vi "水样测试配置.vi"() -> (2 "确认输出":bool, 3 "水样测定时间输出":dbl=1.0)   [LabVIEW 2016, in "斯坦道多参数.lvlib"]
uses:
  <vilib>/Utility/config.llb/NI_LVConfig.lvlib
  <vilib>/Utility/miscctls.llb/LVPointTypeDef.ctl
panel:
  in  "取消":bool
  in  "确定":bool
  in  "水样测试时间":dbl=1.0
  # "请输入水样测定时间"
  # "min"
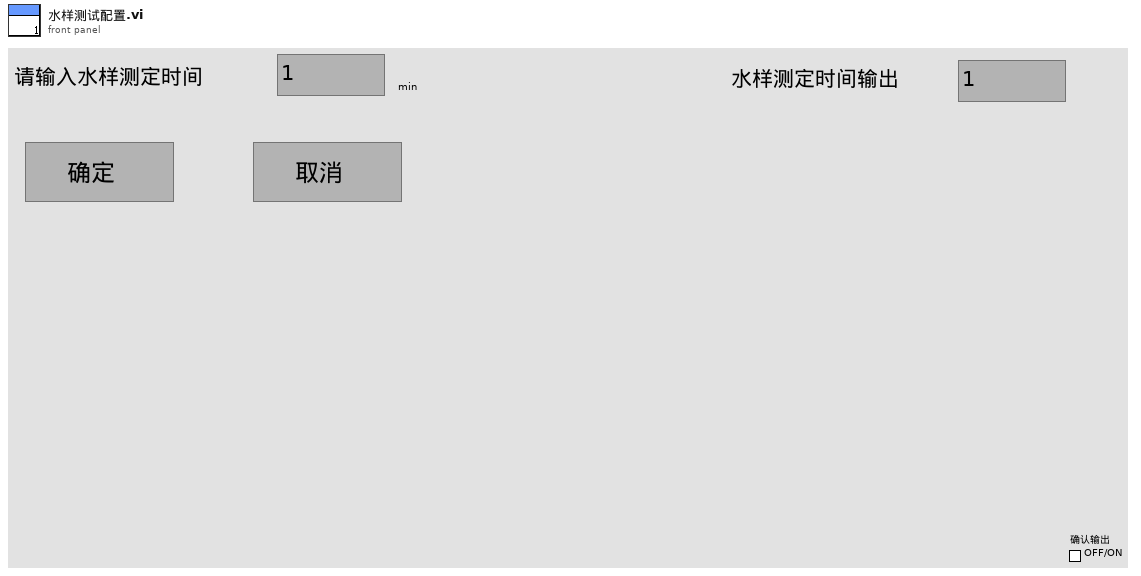
[diagram p1: front panel]
types:
  T1 = typedef "LVPointTypeDef.ctl" = cluster{"Horizontal":i16, "Vertical":i16}
  T2 = typedef "NI_LVConfig.lvlib/Config Data RefNum.ctl" = refnum<k1>
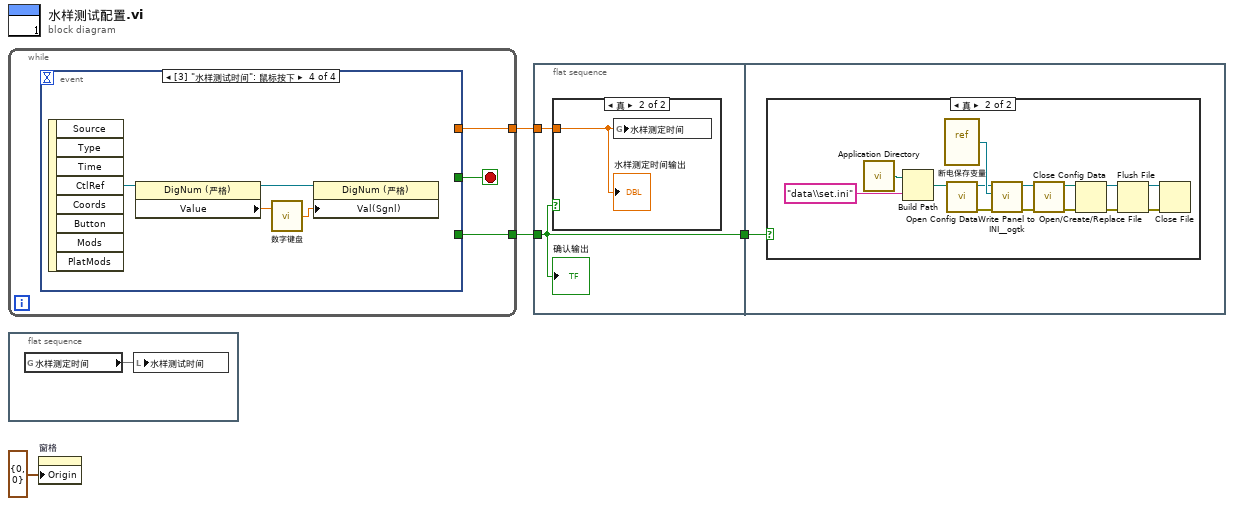
[diagram p0: block diagram]
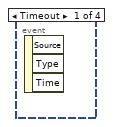
[diagram p4: hidden frame]
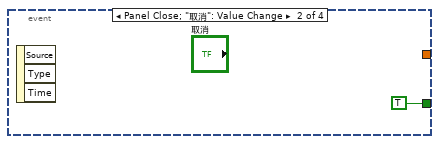
[diagram p5: hidden frame]
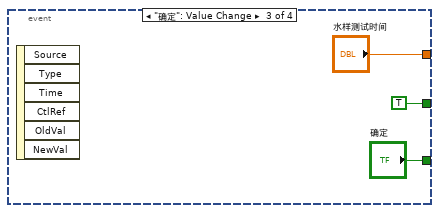
[diagram p6: hidden frame]
diagram:
  n1 = while {
    tunnel: [w6] -> w3
    tunnel: [w5] -> w4
    stop <- w7 stop-if-true
    n2 = event shown="[3] \"水样测试时间\": 鼠标按下" {
      selector: _ -> [_ _ _ _]
      dyn-events: _ -> [_ _ _ _]
      timeout: _ -> [_ _ _ _]
      tunnel: [_ TRUE TRUE _] -> w7
      tunnel: [_ _ "水样测试时间" _] -> w6
      tunnel: [_ _ "确定" _] -> w5
      event Timeout {
        n3 = event-data() -> ()  [unwired: 1 in, 3 out]
      }
      event Panel Close; "取消": Value Change {
        n4 = event-data() -> ()  [unwired: 1 in, 3 out]
      }
      event "确定": Value Change {
        n5 = event-data() -> ()  [unwired: 1 in, 6 out]
      }
      event "水样测试时间": Mouse Down {
        n6 = event-data() -> ("CtlRef"=w15:refnum<vi>)  [unwired: 1 in, 7 out]
        n7 = property class="DigNum (严格)"(reference=w15) -> (reference out=w12:refnum<vi>, "Value"=w14:dbl)  [unwired: 1 in, 1 out]
        n8 = call "数字键盘.vi"("OldNumber"=w14) -> ("NewNumber"=w13:dbl)  [unwired: 1 in]
        n9 = property class="DigNum (严格)"(reference=w12, "Val(Sgnl)"=w13) -> ()  [unwired: 1 in, 2 out]
      }
    }
  }
  n10 = flat-sequence {
    frame #0 {
      n11 = global read "断电保存变量.vi" "水样测定时间"() -> (w16)
      n12 = local write "水样测试时间"(w16) -> ()
    }
  }
  n13 = property on="窗格" class="Pane"("Origin"=T1 {"Horizontal"=0, "Vertical"=0} ("原点")) -> ()  [unwired: 2 in, 2 out]
  n14 = flat-sequence {
    tunnel: w4 -> [w17]
    tunnel: w3 -> [w18]
    tunnel: [w17] -> w2
    tunnel: w2 -> [w20]
    frame #0 {
      n15 = case shown="真" w17 {
        tunnel: w18 -> [_ w19]
        frame False {
        }
        frame True {
          n16 = global write "断电保存变量.vi" "水样测定时间"(w19) -> ()
          "水样测定时间输出" <- w19
        }
      }
      "确认输出" <- w17
    }
    frame #1 {
      n17 = case shown="真" w20 {
        frame False {
        }
        frame True {
          n18 = call <vilib>:"Application Directory.vi"() -> ("Application Directory"=w25:path)
          n19 = Build Path(base path=w25, name or relative path="data\\set.ini" ("名称或相对路径")) -> (appended path=w26:path)
          n20 = vi-ref "断电保存变量.vi"() -> (w28:refnum<vi>)
          n21 = call <vilib>:"Open Config Data.vi"("configuration file path"=w26) -> ("error out"=w22:errorcluster, "refnum"=w21:T2)  [unwired: 8 in, 1 out]
          n22 = call <userlib>:"Write Panel to INI__ogtk.vi"("error in (no error)"=w22, "VI ref"=w28, "refnum"=w21) -> ("error out"=w24:errorcluster, "refnum out"=w23:T2)  [unwired: 7 in]
          n23 = call <vilib>:"Close Config Data.vi"("error in (no error)"=w24, "refnum"=w23) -> ("error out"=w32:errorcluster, "file path"=w31:path)  [unwired: 8 in]
          n24 = Open/Create/Replace File(file path (use dialog)=w31, error in=w32) -> (refnum out=w30:refnum<file>, error out=w29:errorcluster)  [unwired: 4 in, 1 out]
          n25 = Flush File(refnum=w30, error in=w29) -> (refnum out=w34:refnum<file>, error out=w33:errorcluster)
          n26 = Close File(refnum=w34, error in=w33) -> ()  [unwired: 2 out]
        }
      }
    }
  }
